vi "Read Multiple Data Points.vi"(8 "error in (no error)":errorcluster, 10 "Qty":u32, 11 "3446X in":refnum<class "3446X.lvclass">) -> (0 "error out":errorcluster, 2 "Values":dbl[](array[numeric]), 3 "3446X out":refnum<class "3446X.lvclass">)   [LabVIEW 2018, in "3446X.lvlib" / "3446X.lvclass"]
uses:
  3446X.lvclass
  3446X.lvclass/3446X.ctl
  <instrlib>/Agilent 3446X Series/Public/Data/Read (Multiple Points).vi
  <instrlib>/Agilent 3446X Series/Agilent 3446X Series.lvlib
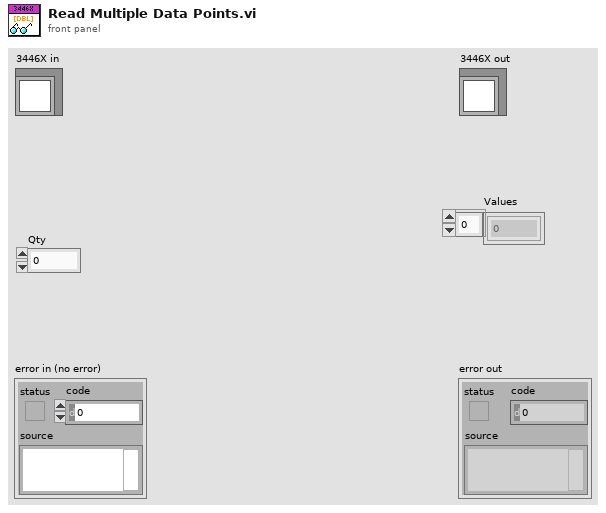
[diagram p1: front panel]
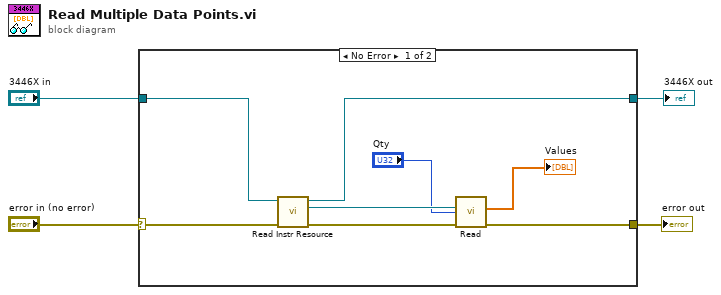
[diagram p0: block diagram]
diagram:
  n1 = case shown="No Error" "error in (no error)" {
    selector: "error in (no error)" -> [w12 w13]
    tunnel: [w8 w14] -> w3
    tunnel: "3446X in" -> [w11 w14]
    tunnel: [w5 w13] -> w1
    frame No Error {
      n2 = call "Read Instr Resource.vi"("error in (no error)"=w12, "3446X in"=w11) -> ("error out"=w10:errorcluster, "Instr Resource"=w9:refnum<visa-resource-name>, "3446X out"=w8:refnum<class "3446X.lvclass">)  [unwired: 7 in]
      n3 = call-poly <instrlib>:"Read.vi"("error in (no error)"=w10, "Sample Count (1)"="Qty", "VISA resource name"=w9) -> ("error out"=w5:errorcluster, "Measurements"=→"Values":dbl[])  [unwired: 6 in, 1 out]
    }
    frame Error {
    }
  }
  "error out" <- w1
  "3446X out" <- w3
